vi "RC Object to RC Enum.vi"(8 "error in (no error)":errorcluster, 11 "RemoteControl in":refnum<class "RemoteControl.lvclass">) -> (0 "error out":errorcluster, 3 "RC Type":T1)   [LabVIEW 2019, in "RemoteControl.lvclass"]
uses:
  RemoteControl.lvclass
  Typedefs/RC Com Type--enum.ctl
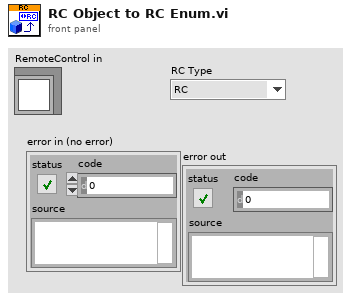
[diagram p1: front panel]
types:
  T1 = typedef "RemoteControl.lvclass/RC Com Type--enum.ctl" = enum16{"RC", "STM", "ZMQ"}
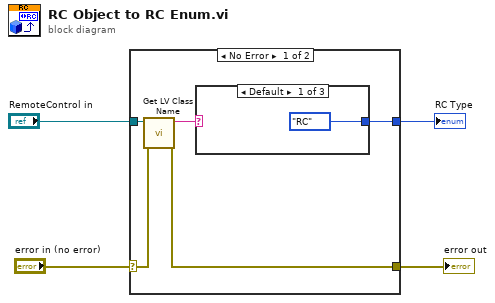
[diagram p0: block diagram]
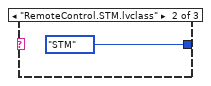
[diagram p2: hidden frame]
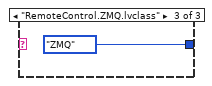
[diagram p3: hidden frame]
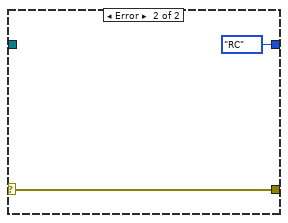
[diagram p4: hidden frame]
diagram:
  n1 = case shown="No Error" "error in (no error)" {
    selector: "error in (no error)" -> [w6 w14]
    tunnel: "RemoteControl in" -> [w9 _]
    tunnel: [w7 RC_Com_Type--enum."RC" ("RC Type")] -> w3
    tunnel: [w5 w14] -> w1
    frame No Error {
      n2 = call <vilib>:"Get LV Class Name.vi"("error in (no error)"=w6, "object"=w9) -> ("error out"=w5:errorcluster, "class name"=w8:string)  [unwired: 8 in]
      n3 = case shown="Default" w8 {
        tunnel: [RC_Com_Type--enum."RC" ("RC Type") RC_Com_Type--enum."STM" ("RC Type") RC_Com_Type--enum."ZMQ" ("RC Type")] -> w7
        frame Default {
        }
        frame "RemoteControl.STM.lvclass" {
        }
        frame "RemoteControl.ZMQ.lvclass" {
        }
      }
    }
    frame Error {
    }
  }
  "RC Type" <- w3
  "error out" <- w1
